vi "U6 6-Counter.vi"() -> ()   [LabVIEW 2021]
panel:
  out "Counter Reads":u32[](array[numeric])
  in  "Timer/Counter Pin Offset":u8
  in  "Reset Counters":bool
  in  "Iteration Inverval (ms)":u32=1000
  out "Timer Value Reads":u32[](array[numeric])
  out "Iteration":i32
  in  "error in":errorcluster
  in  "Address":string="1"
  in  "FirstFound":bool=TRUE
  in  "stop":bool
  out "error out":errorcluster
  out "Error Message":string
  # "Enables all 4 firmware counters (timers) and both hardware counters, then reads\nall at the specified interval.  Timers will be assigned to pins starting with FIO0 plus\npin offset, and the hardware counters will get the next two pins after the timers."
  # "Firmware Counter 0"
  # "Firmware Counter 1"
  # "Firmware Counter 2"
  # "Firmware Counter 3"
  # "Counter 0"
  # "Counter 1"
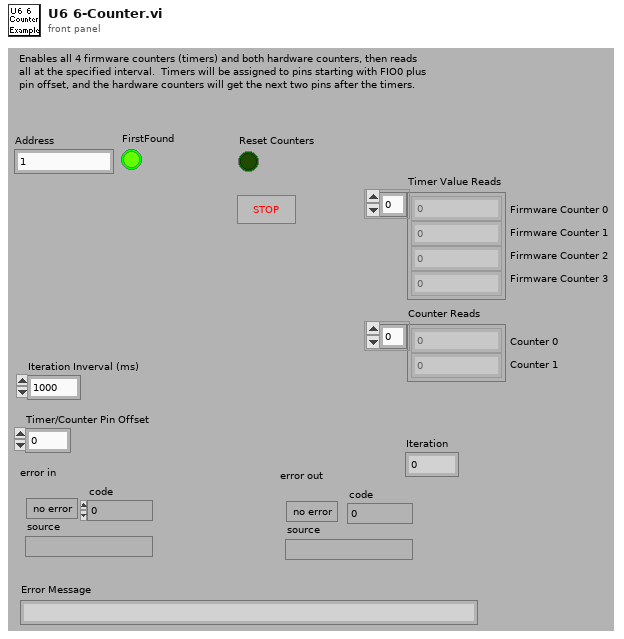
[diagram p1: front panel]
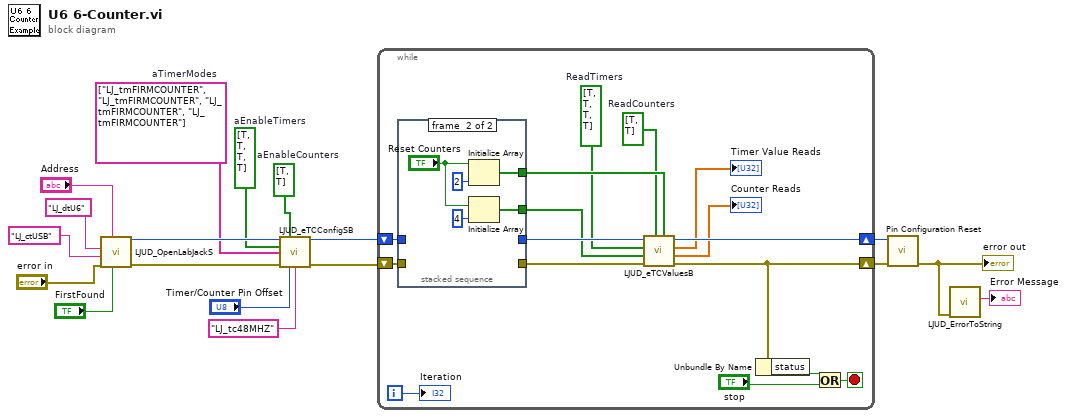
[diagram p0: block diagram]
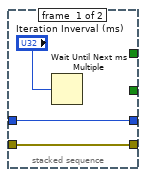
[diagram p2: hidden frame]
diagram:
  w5 = string[] ["LJ_tmFIRMCOUNTER", "LJ_tmFIRMCOUNTER", "LJ_tmFIRMCOUNTER", "LJ_tmFIRMCOUNTER"]  # aTimerModes
  w6 = bool[] [TRUE, TRUE, TRUE, TRUE]  # aEnableTimers
  w7 = bool[] [TRUE, TRUE]  # aEnableCounters
  n1 = call "LJUD_OpenLabJackS.vi"("FirstFound"="FirstFound", "Address"="Address", "error in"="error in", "ConnectionType"="LJ_ctUSB", "DeviceType"="LJ_dtU6") -> ("error out"=w11:errorcluster, "Handle"=w12:i32)  [unwired: 4 in, 1 out]
  n2 = call "LJUD_eTCConfigSB.vi"("Handle In"=w12, "aEnableCounters"=w7, "aEnableTimers"=w6, "aTimerModes"=w5, "error in"=w11, "TCPinOffset"="Timer/Counter Pin Offset", "TimerClockBase"="LJ_tc48MHZ") -> ("Handle Out"=w8:i32, "error out"=w9:errorcluster)  [unwired: 7 in]
  n3 = while {
    shift-left: w9 -> [w33]
    shift-right: [w27] -> w3
    shift-left: w8 -> [w34]
    shift-right: [w26] -> w4
    i -> [w29]
    stop <- w32 stop-if-true
    w20 = bool[] [TRUE, TRUE, TRUE, TRUE]  # ReadTimers
    w23 = bool[] [TRUE, TRUE]  # ReadCounters
    n4 = stacked-sequence {
      tunnel: [w37 _] -> w25
      tunnel: [w36 _] -> w28
      tunnel: w34 -> [w37 _]
      tunnel: w33 -> [w36 _]
      tunnel: [_ w41] -> w24
      tunnel: [_ w38] -> w19
      frame #0 {
        n5 = Wait Until Next ms Multiple(millisecond multiple="Iteration Inverval (ms)") -> ()  [unwired: 1 out]
      }
      frame #1 {
        n6 = Initialize Array("Reset Counters", 2 ("Dimension Size")) -> (w41:bool[])
        n7 = Initialize Array("Reset Counters", 4 ("Dimension Size")) -> (w38:bool[])
      }
    }
    n8 = call "LJUD_eTCValuesB.vi"("aResetCounters"=w24, "aReadCounters"=w23, "error in"=w28, "aUpdateResetTimers"=w19, "aReadTimers"=w20, "Handle In"=w25) -> ("error out"=w27:errorcluster, "aCounterValues"=→"Counter Reads":dbl[], "aTimerValues Read"=→"Timer Value Reads":dbl[], "Handle Out"=w26:i32)  [unwired: 2 in]
    n9 = Unbundle By Name(w27) -> ("status"=w31:bool)
    n10 = Or(x=w31, y="stop") -> (x .or. y?=w32:bool)
    "Iteration" <- w29
  }
  n11 = call "Pin Configuration Reset.vi"("error in"=w3, "Handle In"=w4) -> ("error out"=w2:errorcluster)  [unwired: 8 in, 1 out]
  "error out" <- w2
  n12 = call "LJUD_ErrorToString.vi"("error in"=w2) -> ("String"=→"Error Message":string)  [unwired: 10 in]
